vi "CloseDotNetReference.vi"(1 ".NET Refnum":refnum<k24>) -> (0 "error out":errorcluster)   [LabVIEW 2010]
uses:
  \\camila\f$/Tests/LVBuildValidation/10.0/Automated/FlexLVAdapter30/Refnums/DotNetRefnum/LabviewDNTest.dll
  LabviewDNTest.dll
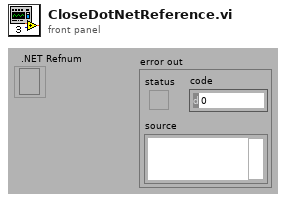
[diagram p1: front panel]
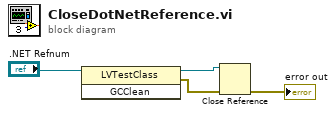
[diagram p0: block diagram]
diagram:
  n1 = invoke class="LVTestClass" method="GCClean"(reference=".NET Refnum") -> (reference out=w2:refnum<k24>, error out=w1:errorcluster)  [unwired: 2 in, 1 out]
  n2 = Close Reference(reference=w2, error in (no error)=w1) -> (error out=→"error out":errorcluster)
